vi "Unix TS to LV (SubVI).vi"(10 "mS":u32, 11 "Unix Time In (s)":u32) -> (3 "Labview Time":timestamp)   [LabVIEW 2019]
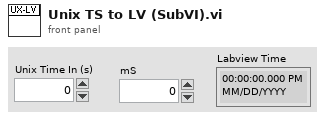
[diagram p1: front panel]
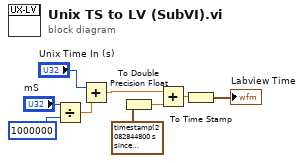
[diagram p0: block diagram]
diagram:
  n1 = Divide(x="mS", y=u32 1000000) -> (x/y=w1:dbl)
  n2 = Add(x="Unix Time In (s)", y=w1) -> (x+y=w4:dbl)
  n3 = To Double Precision Float(number=timestamp(2082844800 s since 1904-01-01)) -> (double precision float=w7:dbl)
  n4 = Add(x=w4, y=w7) -> (x+y=w8:dbl)
  n5 = To Time Stamp(1:w8) -> (0:→"Labview Time":timestamp)
